vi "Validate Custom Device Configuration.vi"(8 "error in (no error)":errorcluster, 9 "Force Validation (F)":bool, 11 "Routing and Faulting Custom Device Ref":T3 format="%.0x") -> (0 "error out":errorcluster, 2 "Module Connection Information":T1[](array[typedef]), 3 "Routing and Faulting Custom Device Ref out":T3 format="%.0x")   [LabVIEW 2020, in "Routing and Faulting System Explorer.lvlib"]
uses:
  Routing and Faulting System Explorer.lvlib
  <vilib>/NI VeriStand/Custom Device API/Custom Device Item Ref.ctl
  Scripting/Types/Module Information.ctl
  Shared/Routing and Faulting Hardware API/Types/Possible Connections for Endpoint.ctl
  Scripting/Validation/Validate From Module Connection Information.vi
  Scripting/Routing and Faulting Scripting.lvlib
  <vilib>/NI VeriStand/Custom Device API/Custom Device API.lvlib
  Shared/Routing and Faulting Hardware API/Routing and Faulting Hardware API.lvlib
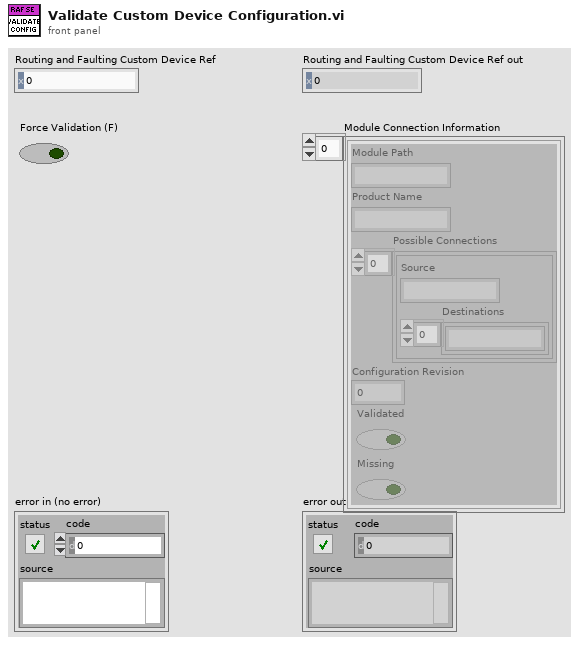
[diagram p1: front panel]
types:
  T1 = typedef "Routing and Faulting Scripting.lvlib/Module Information.ctl" = cluster{"Module Path":string, "Product Name":string, "Possible Connections":T2[], "Configuration Revision":u32, "Validated":bool, "Missing":bool}
  T2 = typedef "Routing and Faulting Hardware API.lvlib/Possible Connections for Endpoint.ctl" = cluster{"Source":string, "Destinations":string[]}
  T3 = typedef "Custom Device API.lvlib/Custom Device Item Ref.ctl" = u64
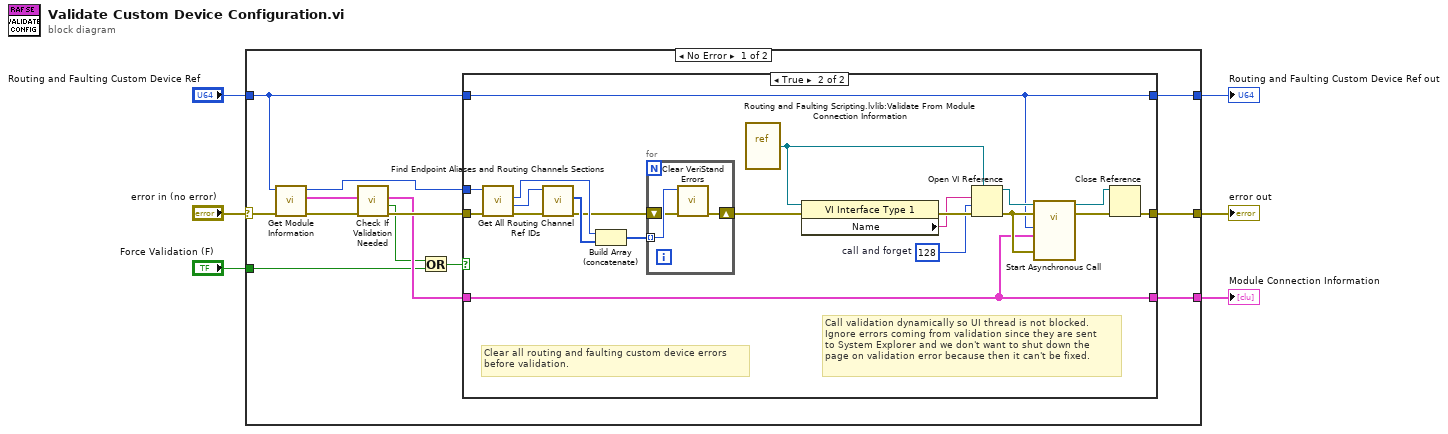
[diagram p0: block diagram]
diagram:
  n1 = case shown="No Error" "error in (no error)" {
    selector: "error in (no error)" -> [w18 w47]
    tunnel: "Routing and Faulting Custom Device Ref" -> [w13 w46]
    tunnel: [w19 w47] -> w5
    tunnel: [w12 w46] -> w3
    tunnel: [w10 _] -> w2
    tunnel: "Force Validation (F)" -> [w9 _]
    frame No Error {
      n2 = call "Get Module Information.vi"("error in"=w18, "routing and faulting in"=w13) -> ("error out"=w17:errorcluster, "module information"=w15:T1[], "routing and faulting out"=w14:T3)  [unwired: 7 in]
      n3 = call "Check If Validation Needed.vi"("error in (no error)"=w17, "Module Information in"=w15) -> ("error out"=w16:errorcluster, "Needs Validation"=w8:bool, "Module Information out"=w11:T1[])  [unwired: 7 in]
      n4 = Or(x=w8, y=w9) -> (x .or. y?=w7:bool)
      n5 = case shown="True" w7 {
        tunnel: [w21 w37] -> w19
        tunnel: w16 -> [w21 w26]
        tunnel: w14 -> [_ w25]
        tunnel: w13 -> [w22 w24]
        tunnel: [w22 w24] -> w12
        tunnel: w11 -> [w20 w23]
        tunnel: [w20 w23] -> w10
        frame False {
        }
        frame True {
          w30 = 128  # call and forget
          # "Call validation dynamically so UI thread is not blocked.\nIgnore errors coming from validation since they are sent\nto System Explorer and we don't want to shut down the\npage on validation error because then it can't be fixed."
          # "Clear all routing and faulting custom device errors\nbefore validation."
          n6 = call "Find Endpoint Aliases and Routing Channels Sections.vi"("error in"=w26, "routing and faulting custom device in"=w25) -> ("error out"=w36:errorcluster, "routing channels"=w35:T3, "endpoint aliases"=w33:T3)  [unwired: 6 in, 1 out]
          n7 = call "Get All Routing Channel Ref IDs.vi"("error in"=w36, "routing channels in"=w35) -> ("error out"=w31:errorcluster, "all routing channels"=w34:T3[])  [unwired: 7 in, 1 out]
          n8 = Build Array (concatenate)(w33, w34) -> (w32:T3[])
          n9 = for {
            tunnel: w32 -> [w44] mode=indexing
            shift-right: [w45] -> w42
            shift-left: w31 -> [w43]
            n10 = call "Clear VeriStand Errors.vi"("error in (no error)"=w43, "Device Item Ref in"=w44) -> ("error out"=w45:errorcluster)  [unwired: 8 in, 1 out]
          }
          n11 = vi-ref "Routing and Faulting Scripting.lvlib:Validate From Module Connection Information.vi"() -> (w29:refnum<vi>)
          n12 = property class="VI Interface Type 1"(reference=w29, error in=w42) -> (error out=w41:errorcluster, "Name"=w40:string)  [unwired: 1 out]
          n13 = Open VI Reference(type specifier VI Refnum (for type only)=w29, vi path=w40, options=w30, error in (no error)=w41) -> (vi reference=w39:refnum<vi>, error out=w38:errorcluster)  [unwired: 2 in]
          n14 = call-by-ref "Start Asynchronous Call"(reference=w39, error in=w38, "error in"=w38, "module connection information in"=w23, "routing and faulting in"=w24) -> (reference out=w27:refnum<vi>, error out=w28:errorcluster)  [unwired: 6 in, 3 out]
          n15 = Close Reference(reference=w27, error in (no error)=w28) -> (error out=w37:errorcluster)
        }
      }
    }
    frame Error {
    }
  }
  "error out" <- w5
  "Routing and Faulting Custom Device Ref out" <- w3
  "Module Connection Information" <- w2
